vi "Calculate Duration.vi"(9 "Sample Rate":i32, 10 "Amplitude":dbl, 11 "Y Values":dbl[](array[numeric])) -> (3 "Duration":dbl)   [LabVIEW 2016, in "Exponential Fit.lvclass"]
uses:
  Exponential Fit.lvclass
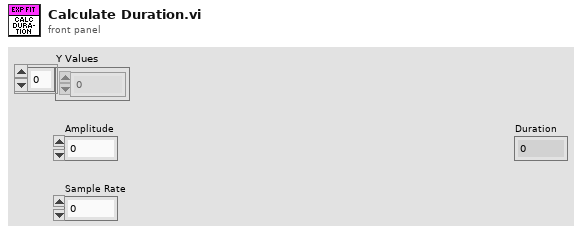
[diagram p1: front panel]
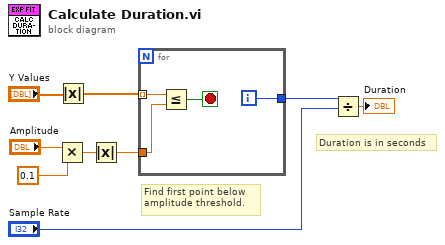
[diagram p0: block diagram]
diagram:
  # "Duration is in seconds"
  # "Find first point below \namplitude threshold."
  n1 = Multiply(x="Amplitude", y=0.1) -> (x*y=w3:dbl)
  n2 = Absolute Value(x="Y Values") -> (abs(x)=w2:dbl[])
  n3 = Absolute Value(x=w3) -> (abs(x)=w1:dbl)
  n4 = for {
    tunnel: w2 -> [w13] mode=indexing
    tunnel: w1 -> [w12]
    tunnel: [w10] -> w7
    i -> [w10]
    stop <- w11 stop-if-true
    n5 = Less Or Equal?(x=w13, y=w12) -> (x <= y?=w11:bool)
  }
  n6 = Divide(x=w7, y="Sample Rate") -> (x/y=→"Duration":dbl)
